vi "Write Value.vi"(8 "error in (no error)":errorcluster, 10 "Value":dbl, 11 "Base in":refnum<class "KDemoBase.lvclass">) -> (0 "error out":errorcluster, 3 "Base out":refnum<class "KDemoBase.lvclass">)   [LabVIEW 2015, in "KDemoBase.lvclass"]
uses:
  KDemoBase.lvclass
  KDemoBase.lvclass/KDemoBase.ctl
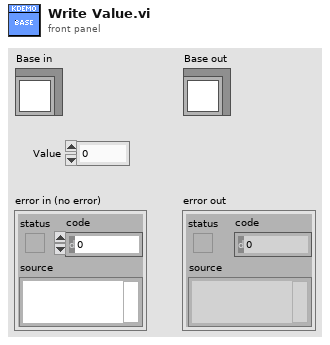
[diagram p1: front panel]
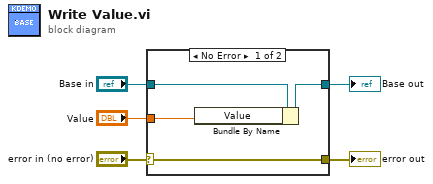
[diagram p0: block diagram]
diagram:
  n1 = case shown="No Error" "error in (no error)" {
    selector: "error in (no error)" -> [w9 w10]
    tunnel: [w9 w10] -> w4
    tunnel: [w7 w11] -> w2
    tunnel: "Base in" -> [w8 w11]
    tunnel: "Value" -> [w6 _]
    frame No Error {
      n2 = Bundle By Name(cluster=w8, "Value"=w6) -> (w7:refnum<class "KDemoBase.lvclass">)
    }
    frame Error {
    }
  }
  "error out" <- w4
  "Base out" <- w2
